vi "set_repetition_rate.vi"(8 "error in (no error)":errorcluster, 10 "repetition rate":dbl[unit], 11 "TrajectoryMH100122AODRAPS in":refnum<class "TrajectoryMH100122AODRAPS.lvclass">) -> (0 "error out":errorcluster, 3 "TrajectoryMH100122AODRAPS out":refnum<class "TrajectoryMH100122AODRAPS.lvclass">)   [LabVIEW 2010, in "TrajectoryMH100122AODRAPS.lvclass"]
doc: "sets the repetition rate in Hz (i.e., repetition/cycles per second)"
uses:
  TrajectoryMH100122AODRAPS.lvclass
  TrajectoryMG100122GenericFPGA/TrajectoryMG100122GenericFPGA/TrajectoryMG100122GenericFPGA.lvclass
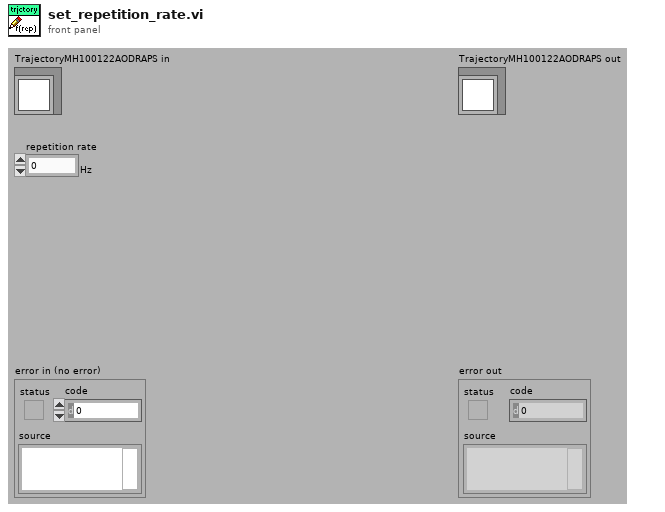
[diagram p1: front panel]
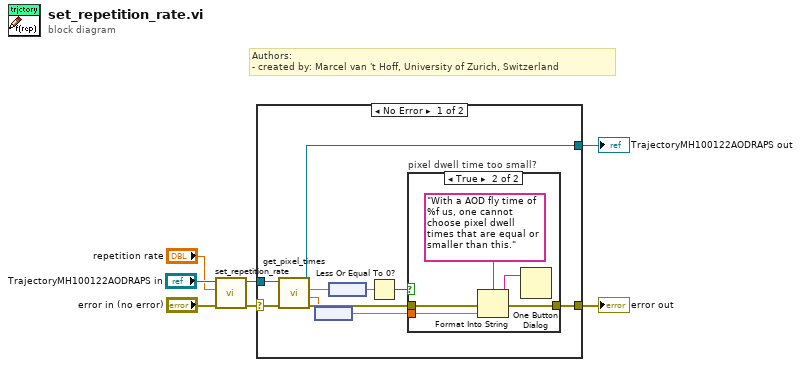
[diagram p0: block diagram]
diagram:
  # "Authors: \n- created by: Marcel van 't Hoff, University of Zurich, Switzerland"
  n1 = call-parent "set_repetition_rate.vi"("error in (no error)"="error in (no error)", "repetition rate"="repetition rate", "GenericTrajectory in"="TrajectoryMH100122AODRAPS in") -> ("error out"=w5:errorcluster, "GenericTrajectory out"=w2:refnum<class "TrajectoryMH100122AODRAPS.lvclass">)  [unwired: 7 in]
  n2 = case shown="No Error" w5 {
    selector: w5 -> [w13 w25]
    tunnel: [w16 w25] -> w4
    tunnel: [w14 w24] -> w3
    tunnel: w2 -> [w15 w24]
    frame No Error {
      n3 = call-dynamic "get_pixel_times.vi"("error in (no error)"=w13, "TrajectoryMG100122AODFrameScan in"=w15) -> ("error out"=w12:errorcluster, "equilibration time"=w9:dbl[unit], "acquisition time"=w11:dbl[unit], "TrajectoryMG100122AODFrameScan out"=w14:refnum<class "TrajectoryMH100122AODRAPS.lvclass">)  [unwired: 5 in, 1 out]
      n4 = node(w9) -> (w8:dbl)
      n5 = node(w11) -> (w10:dbl)
      n6 = Less Or Equal To 0?(x=w10) -> (x <= 0?=w17:bool)
      n7 = case "pixel dwell time too small?" shown="True" w17 {
        tunnel: w12 -> [w18 w23]
        tunnel: [w18 w22] -> w16
        tunnel: w8 -> [_ w21]
        frame False {
        }
        frame True {
          n8 = Format Into String(format string="With a AOD fly time of %f us, one cannot choose pixel dwell times that are equal or smaller than this.", error in=w23, w21) -> (resulting string=w19:string, error out=w22:errorcluster)  [unwired: 1 in]
          n9 = One Button Dialog(message=w19) -> ()  [unwired: 1 in, 1 out]
        }
      }
    }
    frame Error {
    }
  }
  "error out" <- w4
  "TrajectoryMH100122AODRAPS out" <- w3
